vi "Configure Power Measurement List Single Parameter Set.vi"(7 "Parameter Set (0)":i32, 8 "error in (no error)":errorcluster, 9 "Index (10)":i32=10, 10 "Instance (1)":i32=1, 11 "VISA resource name":refnum<visa-resource-name>) -> (0 "error out":errorcluster, 3 "VISA resource name out":refnum<visa-resource-name>)   [LabVIEW 2020, in "Rohde&Schwarz CMXP GPRF.lvlib"]
doc: "Selects the parameter set for a particular frequency/level step.\n\nAttribute:\nRSCMXPGPRF_ATTR_POWER_MEASUREMENT_LIST_SINGLE_PARAMETER_SET\n\nRemote-control command:\nCONFigure:GPRF:MEAS<i>:POWer:LIST:PSET"
uses:
  <instrlib>/Rohde&Schwarz CMXP GPRF/Rohde&Schwarz CMXP GPRF.lvlib
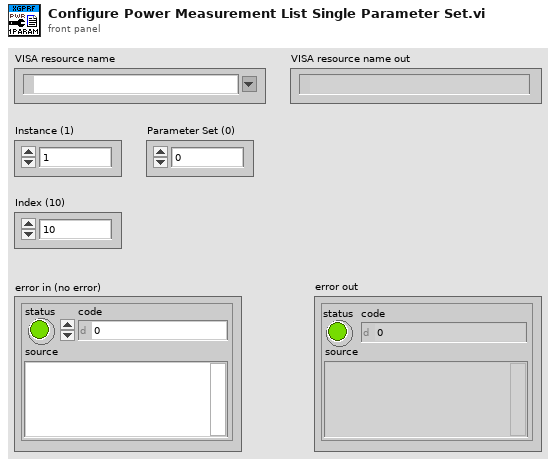
[diagram p1: front panel]
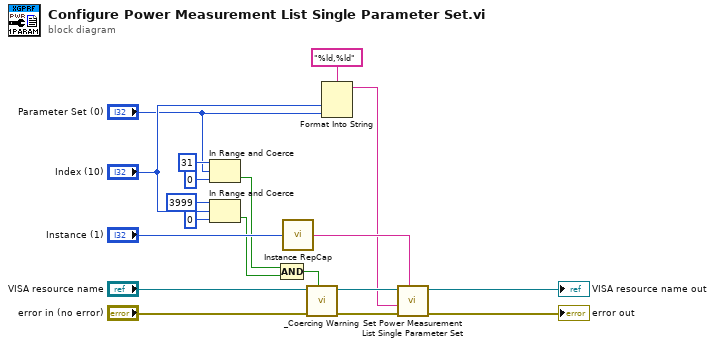
[diagram p0: block diagram]
diagram:
  n1 = In Range and Coerce(upper limit=31, x="Parameter Set (0)", lower limit=0) -> (In Range?=w2:bool)  [unwired: 1 out]
  n2 = In Range and Coerce(upper limit=3999, x="Index (10)", lower limit=0) -> (In Range?=w3:bool)  [unwired: 1 out]
  n3 = Compound Arithmetic op=AND(w2, w3) -> (w12:bool)
  n4 = call <instrlib>:"Instance RepCap.vi"("Instance in"="Instance (1)") -> ("Instance out"=w5:string)
  n5 = call <instrlib>:"_Coercing Warning.vi"("In Range?"=w12, "error in (no error)"="error in (no error)", "VISA resource name"="VISA resource name") -> ("error out"=w9:errorcluster, "VISA resource name out"=w8:refnum<visa-resource-name>)  [unwired: 7 in]
  n6 = Format Into String(format string="%ld,%ld", "Index (10)", "Parameter Set (0)") -> (resulting string=w1:string)  [unwired: 2 in, 1 out]
  n7 = call "Set Power Measurement List Single Parameter Set"("Repeated Capabilities"=w5, "error in (no error)"=w9, "Power Measurement List Single Parameter Set ()"=w1, "instrument handle"=w8) -> ("error out"=→"error out":errorcluster, "instrument handle out"=→"VISA resource name out":refnum<visa-resource-name>)  [unwired: 6 in]
